vi "myRIO_BRig_RT_dataMTrig_main__v2.vi"(0 "input_dataMTrig":u16[](array[numeric]), 2 "input_Audio_trig_L":bool, 3 "input_Audio_trig_R":bool, 5 "input_Laser_trig":bool) -> (14 "output_dataMTrig":u16[](array[numeric]), 16 "output_Audio_L":bool, 17 "output_Audio_R":bool, 19 "output_Laser":bool)   [LabVIEW 2014]
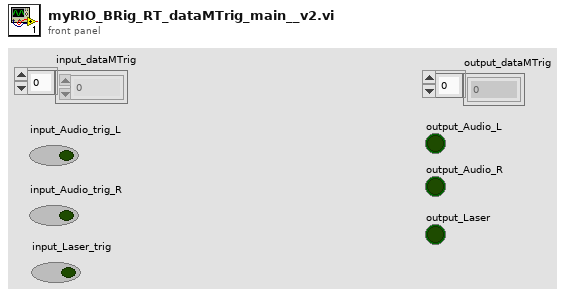
[diagram p1: front panel]
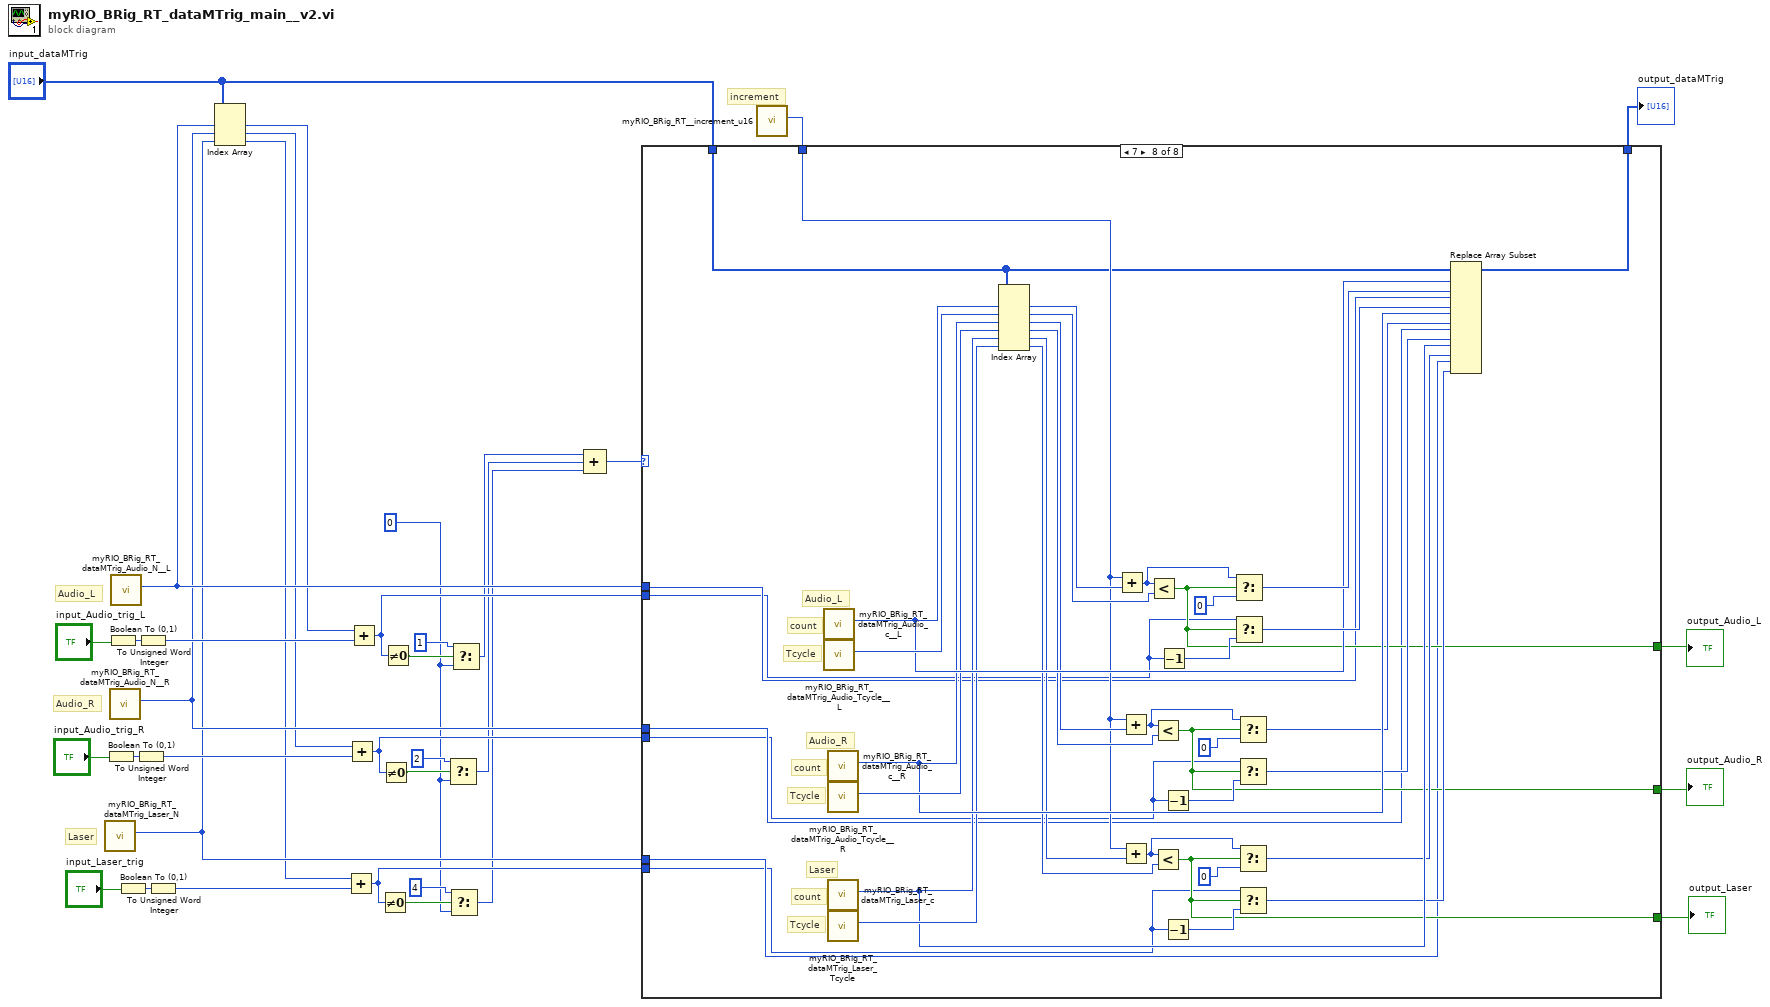
[diagram p0: block diagram]
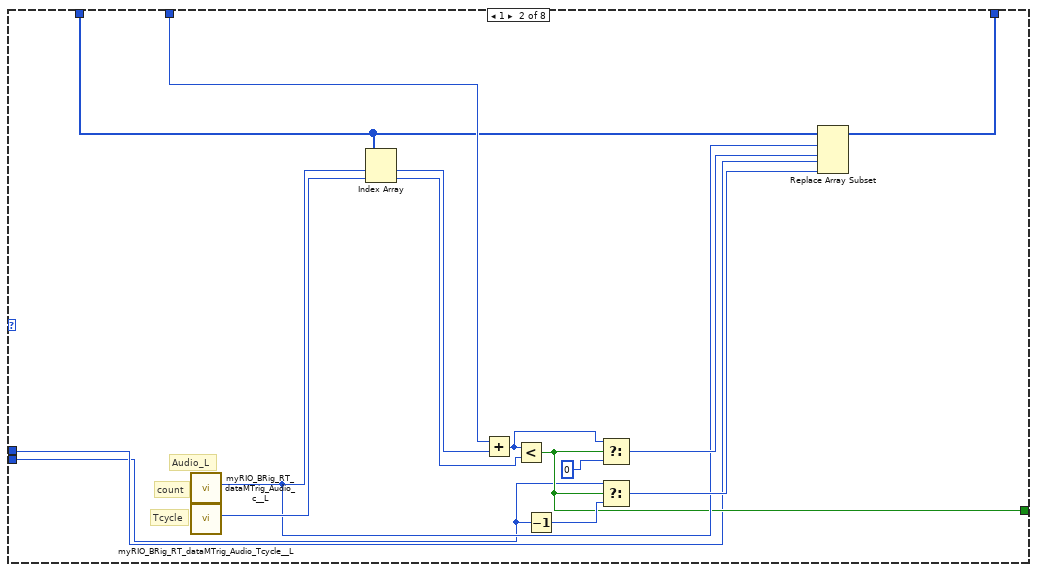
[diagram p3: hidden frame]
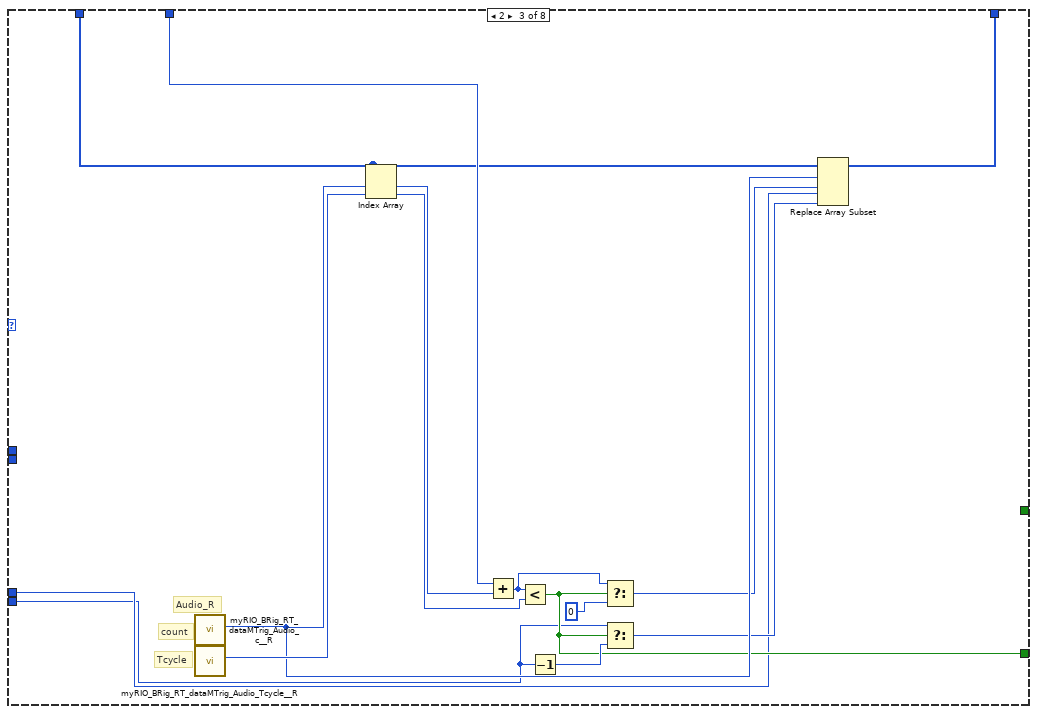
[diagram p4: hidden frame]
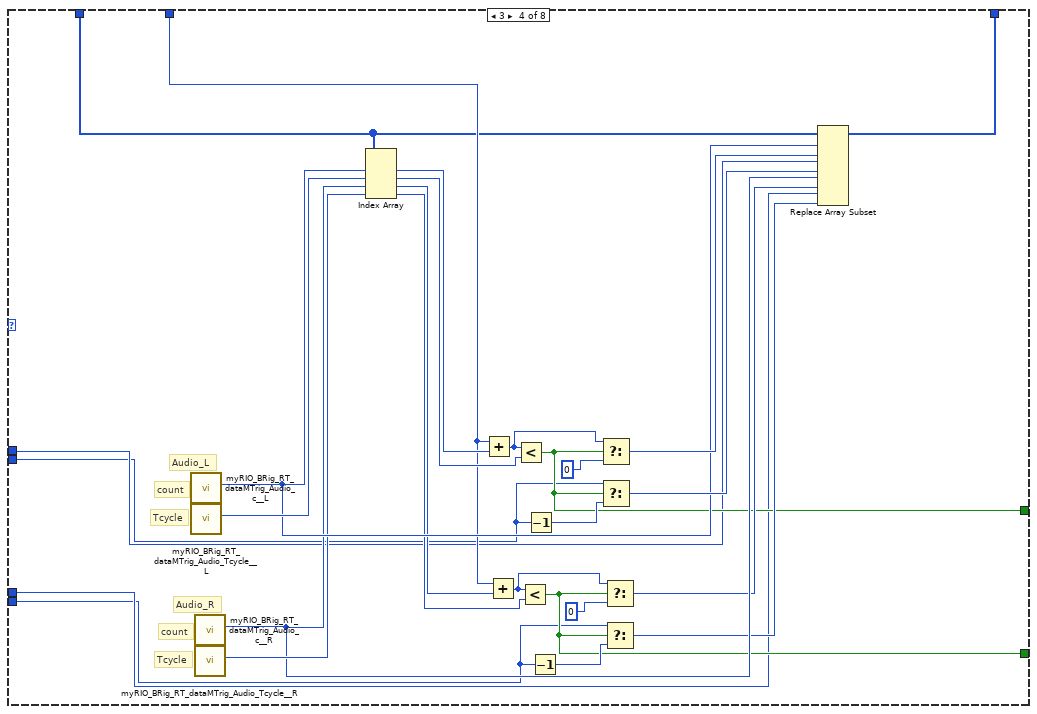
[diagram p5: hidden frame]
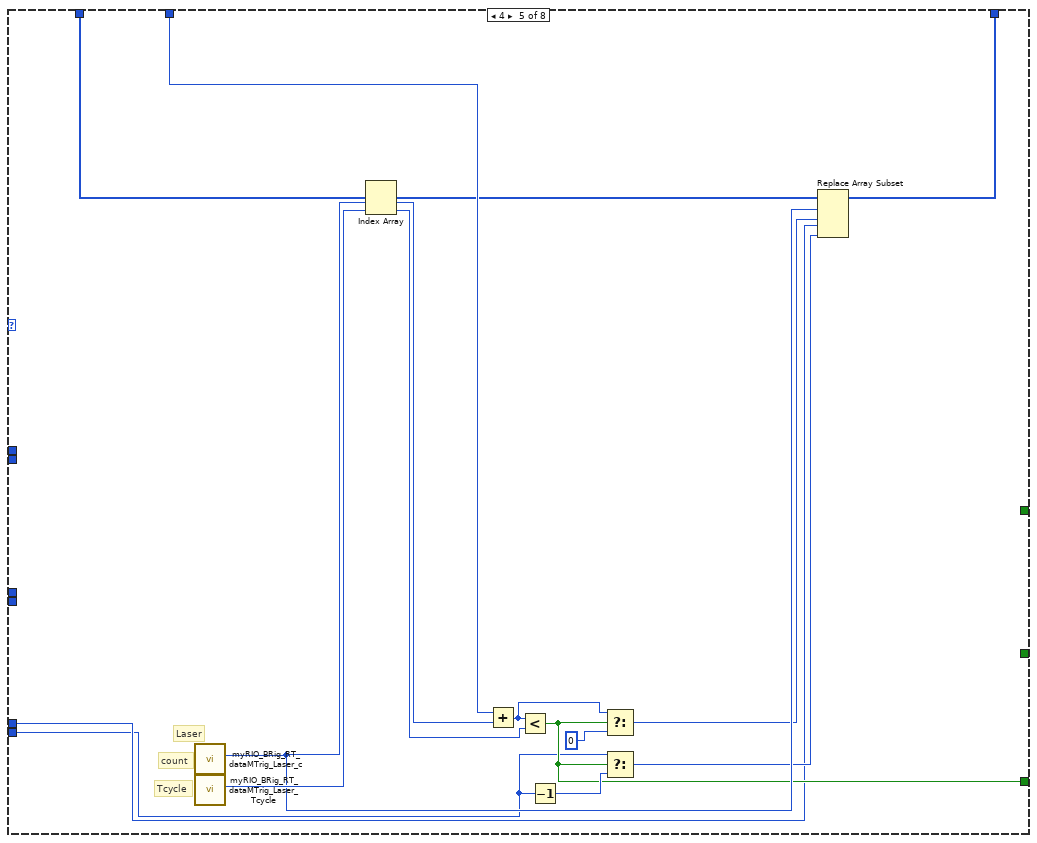
[diagram p6: hidden frame]
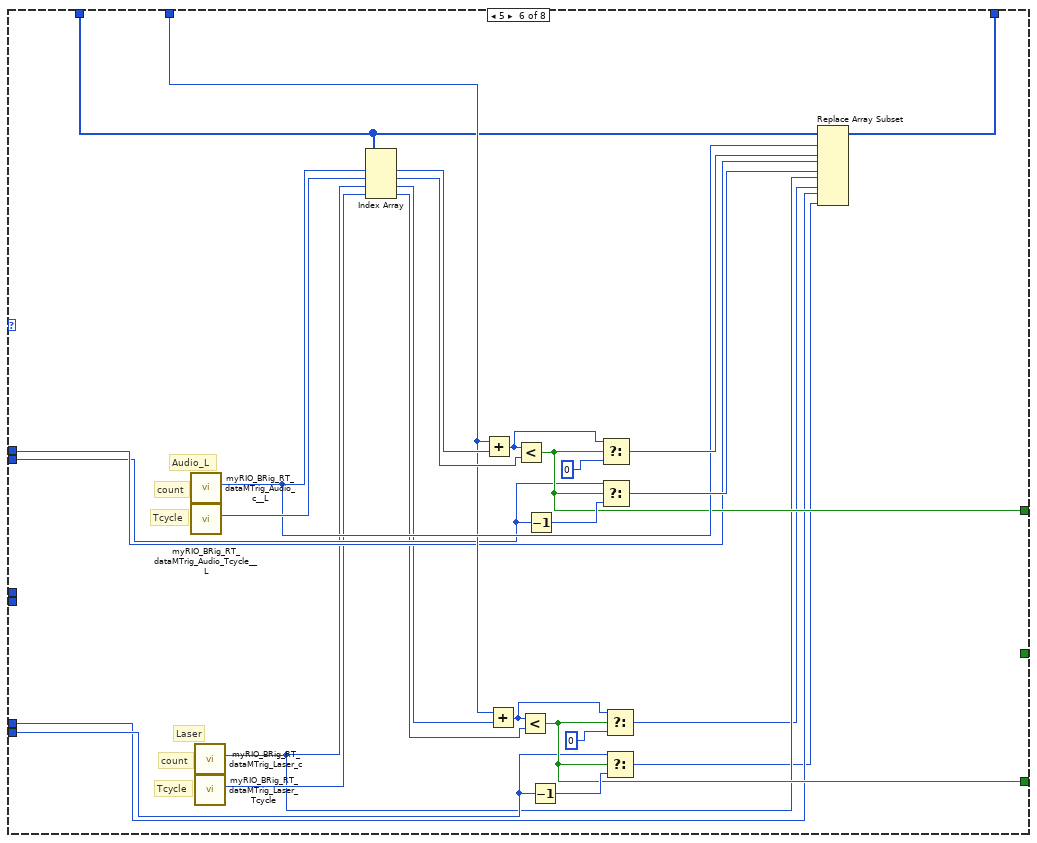
[diagram p7: hidden frame]
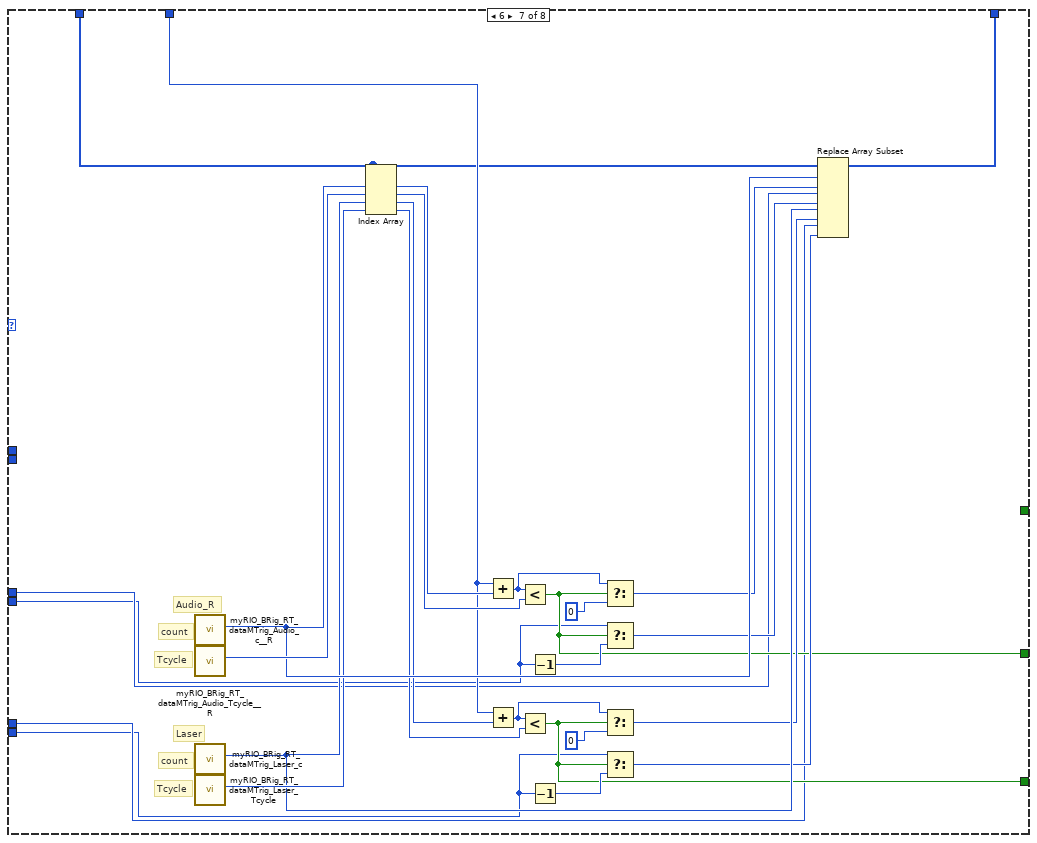
[diagram p8: hidden frame]
diagram:
  w6 = u8 0 ("f")
  # "Laser"
  # "Audio_R"
  # "increment"
  # "Audio_L"
  n1 = call "myRIO_BRig_RT_dataMTrig_Laser_N.vi"() -> ("output_Laser_N"=w7:i32)  [unwired: 11 in]
  n2 = Boolean To (0,1)(Boolean="input_Audio_trig_R") -> (0, 1=w23:i16)
  n3 = Boolean To (0,1)(Boolean="input_Audio_trig_L") -> (0, 1=w35:i16)
  n4 = call "myRIO_BRig_RT_dataMTrig_Audio_N__R.vi"() -> ("output_Audio_N__R"=w17:i32)  [unwired: 11 in]
  n5 = call "myRIO_BRig_RT_dataMTrig_Audio_N__L.vi"() -> ("output_Audio_N__L"=w18:i32)  [unwired: 11 in]
  n6 = Boolean To (0,1)(Boolean="input_Laser_trig") -> (0, 1=w13:i16)
  n7 = To Unsigned Word Integer(number=w23) -> (unsigned 16bit integer=w22:u16)
  n8 = To Unsigned Word Integer(number=w35) -> (unsigned 16bit integer=w34:u16)
  n9 = To Unsigned Word Integer(number=w13) -> (unsigned 16bit integer=w11:u16)
  n10 = Index Array(array="input_dataMTrig", index #1=w18, index #2=w17, index #3=w7) -> (element #1=w16:u16, element #2=w15:u16, element #3=w5:u16)
  n11 = Add(x=w5, y=w11) -> (x+y=w8:u16)
  n12 = Add(x=w15, y=w22) -> (x+y=w19:u16)
  n13 = Add(x=w16, y=w34) -> (x+y=w27:u16)
  n14 = Not Equal To 0?(x=w8) -> (x != 0?=w9:bool)
  n15 = Not Equal To 0?(x=w19) -> (x != 0?=w20:bool)
  n16 = Not Equal To 0?(x=w27) -> (x != 0?=w32:bool)
  n17 = Select(t=u8 2, s=w20, f=w6) -> (s? t:f=w3:u8)
  n18 = Select(t=u8 4, s=w9, f=w6) -> (s? t:f=w2:u8)
  n19 = Select(t=u8 1, s=w32, f=w6) -> (s? t:f=w4:u8)
  n20 = Compound Arithmetic op=ADD(w4, w3, w2) -> (w1:u8)
  n21 = call "myRIO_BRig_RT__increment_u16.vi"() -> ("output_increment__u16"=w30:u16)  [unwired: 11 in]
  n22 = case shown="7" w1 {
    tunnel: "input_dataMTrig" -> [w36 w41 w56 w74 w98 w122 w143 w173]
    tunnel: w30 -> [_ w42 w57 w75 w99 w123 w144 w174]
    tunnel: [w36 w40 w55 w73 w97 w121 w142 w172] -> w29
    tunnel: w18 -> [_ w38 _ w70 _ w118 _ w168]
    tunnel: w27 -> [_ w37 _ w69 _ w117 _ w167]
    tunnel: [_ w39 _ w72 _ w120 _ w171] -> w26
    tunnel: [_ _ w54 w71 _ _ w141 w170] -> w25
    tunnel: [_ _ _ _ w96 w119 w140 w169] -> w24
    tunnel: w17 -> [_ _ w53 w68 _ _ w139 w166]
    tunnel: w19 -> [_ _ w52 w67 _ _ w138 w165]
    tunnel: w7 -> [_ _ _ _ w95 w110 w137 w164]
    tunnel: w8 -> [_ _ _ _ w94 w116 w136 w163]
    frame 0, Default {
    }
    frame 1 {
      # "Audio_L"
      # "Tcycle"
      # "count"
      n23 = call "myRIO_BRig_RT_dataMTrig_Audio_c__L.vi"() -> ("output_Audio_c__L"=w43:i32)  [unwired: 11 in]
      n24 = call "myRIO_BRig_RT_dataMTrig_Audio_Tcycle__L.vi"() -> ("output_Audio_Tcycle__L"=w48:i32)  [unwired: 11 in]
      n25 = Index Array(array=w41, index #1=w43, index #2=w48) -> (element #1=w47:u16, element #2=w46:u16)
      n26 = Add(x=w42, y=w47) -> (x+y=w50:u16)
      n27 = Less?(x=w50, y=w46) -> (x < y?=w39:bool)
      n28 = Decrement(x=w37) -> (x-1=w51:u16)
      n29 = Select(t=w50, s=w39, f=u16 0) -> (s? t:f=w45:u16)
      n30 = Select(t=w37, s=w39, f=w51) -> (s? t:f=w44:u16)
      n31 = Replace Array Subset(array=w41, new element #1=w45, index #1=w43, new element #2=w44, index #2=w38) -> (w40:u16[])
    }
    frame 2 {
      # "Audio_R"
      # "Tcycle"
      # "count"
      n32 = call "myRIO_BRig_RT_dataMTrig_Audio_c__R.vi"() -> ("output_Audio_c__R"=w60:i32)  [unwired: 11 in]
      n33 = call "myRIO_BRig_RT_dataMTrig_Audio_Tcycle__R.vi"() -> ("output_Audio_Tcycle__R"=w61:i32)  [unwired: 11 in]
      n34 = Index Array(array=w56, index #1=w60, index #2=w61) -> (element #1=w63:u16, element #2=w62:u16)
      n35 = Add(x=w57, y=w63) -> (x+y=w65:u16)
      n36 = Less?(x=w65, y=w62) -> (x < y?=w54:bool)
      n37 = Decrement(x=w52) -> (x-1=w66:u16)
      n38 = Select(t=w65, s=w54, f=u16 0) -> (s? t:f=w59:u16)
      n39 = Select(t=w52, s=w54, f=w66) -> (s? t:f=w58:u16)
      n40 = Replace Array Subset(array=w56, new element #1=w59, index #1=w60, new element #2=w58, index #2=w53) -> (w55:u16[])
    }
    frame 3 {
      # "Audio_R"
      # "Tcycle"
      # "count"
      # "Audio_L"
      # "Tcycle"
      # "count"
      n41 = call "myRIO_BRig_RT_dataMTrig_Audio_c__L.vi"() -> ("output_Audio_c__L"=w85:i32)  [unwired: 11 in]
      n42 = call "myRIO_BRig_RT_dataMTrig_Audio_Tcycle__L.vi"() -> ("output_Audio_Tcycle__L"=w90:i32)  [unwired: 11 in]
      n43 = call "myRIO_BRig_RT_dataMTrig_Audio_c__R.vi"() -> ("output_Audio_c__R"=w78:i32)  [unwired: 11 in]
      n44 = call "myRIO_BRig_RT_dataMTrig_Audio_Tcycle__R.vi"() -> ("output_Audio_Tcycle__R"=w79:i32)  [unwired: 11 in]
      n45 = Index Array(array=w74, index #1=w85, index #2=w90, index #3=w78, index #4=w79) -> (element #1=w89:u16, element #2=w88:u16, element #3=w81:u16, element #4=w80:u16)
      n46 = Add(x=w75, y=w89) -> (x+y=w92:u16)
      n47 = Add(x=w75, y=w81) -> (x+y=w83:u16)
      n48 = Less?(x=w92, y=w88) -> (x < y?=w72:bool)
      n49 = Less?(x=w83, y=w80) -> (x < y?=w71:bool)
      n50 = Decrement(x=w69) -> (x-1=w93:u16)
      n51 = Decrement(x=w67) -> (x-1=w84:u16)
      n52 = Select(t=w92, s=w72, f=u16 0) -> (s? t:f=w87:u16)
      n53 = Select(t=w69, s=w72, f=w93) -> (s? t:f=w86:u16)
      n54 = Select(t=w83, s=w71, f=u16 0) -> (s? t:f=w77:u16)
      n55 = Select(t=w67, s=w71, f=w84) -> (s? t:f=w76:u16)
      n56 = Replace Array Subset(array=w74, new element #1=w87, index #1=w85, new element #2=w86, index #2=w70, new element #3=w77, index #3=w78, new element #4=w76, index #4=w68) -> (w73:u16[])
    }
    frame 4 {
      # "Laser"
      # "Tcycle"
      # "count"
      n57 = call "myRIO_BRig_RT_dataMTrig_Laser_c.vi"() -> ("output_Laser_c"=w102:i32)  [unwired: 11 in]
      n58 = call "myRIO_BRig_RT_dataMTrig_Laser_Tcycle.vi"() -> ("output_Laser_Tcycle"=w105:i32)  [unwired: 11 in]
      n59 = Index Array(array=w98, index #1=w102, index #2=w105) -> (element #1=w104:u16, element #2=w103:u16)
      n60 = Add(x=w99, y=w104) -> (x+y=w107:u16)
      n61 = Less?(x=w107, y=w103) -> (x < y?=w96:bool)
      n62 = Decrement(x=w94) -> (x-1=w108:u16)
      n63 = Select(t=w107, s=w96, f=u16 0) -> (s? t:f=w101:u16)
      n64 = Select(t=w94, s=w96, f=w108) -> (s? t:f=w100:u16)
      n65 = Replace Array Subset(array=w98, new element #1=w101, index #1=w102, new element #2=w100, index #2=w95) -> (w97:u16[])
    }
    frame 5 {
      # "Laser"
      # "Tcycle"
      # "count"
      # "Audio_L"
      # "Tcycle"
      # "count"
      n66 = call "myRIO_BRig_RT_dataMTrig_Audio_c__L.vi"() -> ("output_Audio_c__L"=w127:i32)  [unwired: 11 in]
      n67 = call "myRIO_BRig_RT_dataMTrig_Audio_Tcycle__L.vi"() -> ("output_Audio_Tcycle__L"=w132:i32)  [unwired: 11 in]
      n68 = call "myRIO_BRig_RT_dataMTrig_Laser_c.vi"() -> ("output_Laser_c"=w112:i32)  [unwired: 11 in]
      n69 = call "myRIO_BRig_RT_dataMTrig_Laser_Tcycle.vi"() -> ("output_Laser_Tcycle"=w115:i32)  [unwired: 11 in]
      n70 = Index Array(array=w122, index #1=w127, index #2=w132, index #3=w112, index #4=w115) -> (element #1=w131:u16, element #2=w130:u16, element #3=w114:u16, element #4=w113:u16)
      n71 = Add(x=w123, y=w131) -> (x+y=w134:u16)
      n72 = Add(x=w123, y=w114) -> (x+y=w125:u16)
      n73 = Less?(x=w134, y=w130) -> (x < y?=w120:bool)
      n74 = Less?(x=w125, y=w113) -> (x < y?=w119:bool)
      n75 = Decrement(x=w117) -> (x-1=w135:u16)
      n76 = Decrement(x=w116) -> (x-1=w126:u16)
      n77 = Select(t=w134, s=w120, f=u16 0) -> (s? t:f=w129:u16)
      n78 = Select(t=w117, s=w120, f=w135) -> (s? t:f=w128:u16)
      n79 = Select(t=w125, s=w119, f=u16 0) -> (s? t:f=w111:u16)
      n80 = Select(t=w116, s=w119, f=w126) -> (s? t:f=w109:u16)
      n81 = Replace Array Subset(array=w122, new element #1=w129, index #1=w127, new element #2=w128, index #2=w118, new element #3=w111, index #3=w112, new element #4=w109, index #4=w110) -> (w121:u16[])
    }
    frame 6 {
      # "Laser"
      # "Tcycle"
      # "count"
      # "Audio_R"
      # "Tcycle"
      # "count"
      n82 = call "myRIO_BRig_RT_dataMTrig_Audio_c__R.vi"() -> ("output_Audio_c__R"=w156:i32)  [unwired: 11 in]
      n83 = call "myRIO_BRig_RT_dataMTrig_Audio_Tcycle__R.vi"() -> ("output_Audio_Tcycle__R"=w157:i32)  [unwired: 11 in]
      n84 = call "myRIO_BRig_RT_dataMTrig_Laser_c.vi"() -> ("output_Laser_c"=w147:i32)  [unwired: 11 in]
      n85 = call "myRIO_BRig_RT_dataMTrig_Laser_Tcycle.vi"() -> ("output_Laser_Tcycle"=w150:i32)  [unwired: 11 in]
      n86 = Index Array(array=w143, index #1=w156, index #2=w157, index #3=w147, index #4=w150) -> (element #1=w159:u16, element #2=w158:u16, element #3=w149:u16, element #4=w148:u16)
      n87 = Add(x=w144, y=w159) -> (x+y=w161:u16)
      n88 = Add(x=w144, y=w149) -> (x+y=w152:u16)
      n89 = Less?(x=w161, y=w158) -> (x < y?=w141:bool)
      n90 = Less?(x=w152, y=w148) -> (x < y?=w140:bool)
      n91 = Decrement(x=w138) -> (x-1=w162:u16)
      n92 = Decrement(x=w136) -> (x-1=w153:u16)
      n93 = Select(t=w161, s=w141, f=u16 0) -> (s? t:f=w155:u16)
      n94 = Select(t=w138, s=w141, f=w162) -> (s? t:f=w154:u16)
      n95 = Select(t=w152, s=w140, f=u16 0) -> (s? t:f=w146:u16)
      n96 = Select(t=w136, s=w140, f=w153) -> (s? t:f=w145:u16)
      n97 = Replace Array Subset(array=w143, new element #1=w155, index #1=w156, new element #2=w154, index #2=w139, new element #3=w146, index #3=w147, new element #4=w145, index #4=w137) -> (w142:u16[])
    }
    frame 7 {
      # "Laser"
      # "Tcycle"
      # "count"
      # "Audio_R"
      # "Tcycle"
      # "count"
      # "Audio_L"
      # "Tcycle"
      # "count"
      n98 = call "myRIO_BRig_RT_dataMTrig_Audio_c__L.vi"() -> ("output_Audio_c__L"=w193:i32)  [unwired: 11 in]
      n99 = call "myRIO_BRig_RT_dataMTrig_Audio_Tcycle__L.vi"() -> ("output_Audio_Tcycle__L"=w198:i32)  [unwired: 11 in]
      n100 = call "myRIO_BRig_RT_dataMTrig_Audio_c__R.vi"() -> ("output_Audio_c__R"=w186:i32)  [unwired: 11 in]
      n101 = call "myRIO_BRig_RT_dataMTrig_Audio_Tcycle__R.vi"() -> ("output_Audio_Tcycle__R"=w187:i32)  [unwired: 11 in]
      n102 = call "myRIO_BRig_RT_dataMTrig_Laser_c.vi"() -> ("output_Laser_c"=w177:i32)  [unwired: 11 in]
      n103 = call "myRIO_BRig_RT_dataMTrig_Laser_Tcycle.vi"() -> ("output_Laser_Tcycle"=w180:i32)  [unwired: 11 in]
      n104 = Index Array(array=w173, index #1=w193, index #2=w198, index #3=w186, index #4=w187, index #5=w177, index #6=w180) -> (element #1=w197:u16, element #2=w196:u16, element #3=w189:u16, element #4=w188:u16, element #5=w179:u16, element #6=w178:u16)
      n105 = Add(x=w174, y=w197) -> (x+y=w200:u16)
      n106 = Add(x=w174, y=w189) -> (x+y=w191:u16)
      n107 = Add(x=w174, y=w179) -> (x+y=w182:u16)
      n108 = Less?(x=w200, y=w196) -> (x < y?=w171:bool)
      n109 = Less?(x=w191, y=w188) -> (x < y?=w170:bool)
      n110 = Less?(x=w182, y=w178) -> (x < y?=w169:bool)
      n111 = Decrement(x=w167) -> (x-1=w201:u16)
      n112 = Decrement(x=w165) -> (x-1=w192:u16)
      n113 = Decrement(x=w163) -> (x-1=w183:u16)
      n114 = Select(t=w200, s=w171, f=u16 0) -> (s? t:f=w195:u16)
      n115 = Select(t=w167, s=w171, f=w201) -> (s? t:f=w194:u16)
      n116 = Select(t=w191, s=w170, f=u16 0) -> (s? t:f=w185:u16)
      n117 = Select(t=w165, s=w170, f=w192) -> (s? t:f=w184:u16)
      n118 = Select(t=w182, s=w169, f=u16 0) -> (s? t:f=w176:u16)
      n119 = Select(t=w163, s=w169, f=w183) -> (s? t:f=w175:u16)
      n120 = Replace Array Subset(array=w173, new element #1=w195, index #1=w193, new element #2=w194, index #2=w168, new element #3=w185, index #3=w186, new element #4=w184, index #4=w166, new element #5=w176, index #5=w177, new element #6=w175, index #6=w164) -> (w172:u16[])
    }
  }
  "output_dataMTrig" <- w29
  "output_Audio_L" <- w26
  "output_Audio_R" <- w25
  "output_Laser" <- w24
